vi "Slide.vi"(7 "Name (\"\" to Use UUID)":string="Event CSM") -> ()   [LabVIEW 2020]
uses:
  <userlib>/_NEVSTOP/Communicable State Machine(CSM)/AdvanceAPI/CSM - Revert Arguments-Safe String.vi
  <userlib>/_NEVSTOP/Communicable State Machine(CSM)/_Shared/Trim Single-line Text.vi
  <userlib>/_NEVSTOP/Communicable State Machine(CSM)/AdvanceAPI/CSM - Make String Arguments Safe.vi
  <userlib>/_NEVSTOP/Communicable State Machine(CSM)/AdvanceAPI/CSM - Break Down Multiple States String.vi
  <userlib>/_NEVSTOP/Communicable State Machine(CSM)/AdvanceAPI/CSM - Compact Multiple States.vi
  <userlib>/_NEVSTOP/Communicable State Machine(CSM)/AdvanceAPI/CSM - Keywords.vi
  <userlib>/_NEVSTOP/Communicable State Machine(CSM)/Communicable State Machine.lvlib
panel:
  out "Slide":u8(slide) scale=0.0..100.0
  out "State History":string
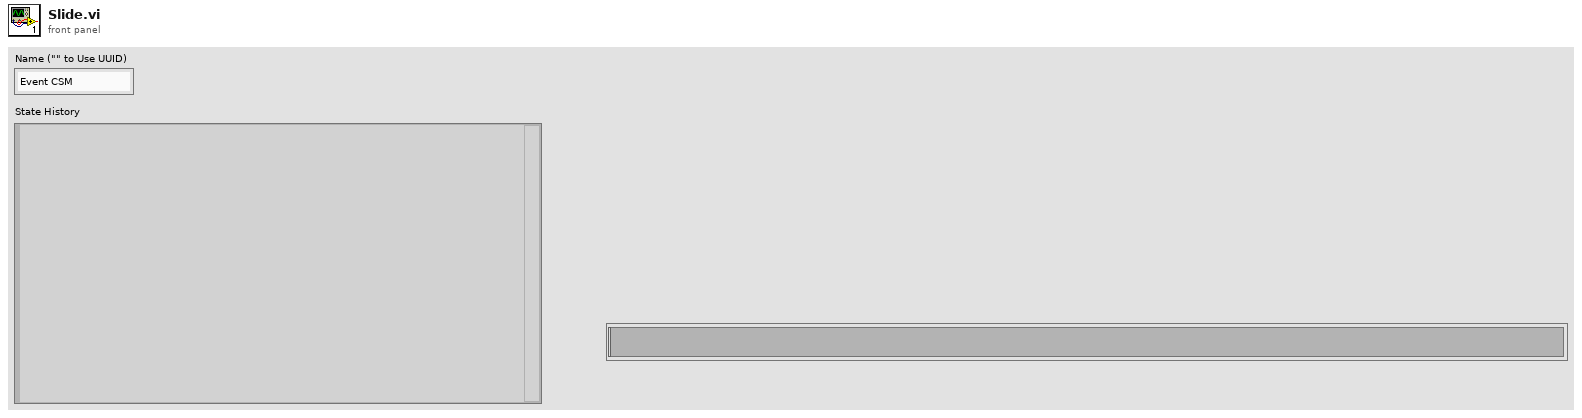
[diagram p1: front panel]
types:
  T1 = enum32{"Invalid", "Standard", "Closed", "Hidden", "Minimized", "Maximized"}
  T2 = enum32{"invalid app kind", "Development System", "Run Time System", "Student Edition", "Embedded LabVIEW", "Evaluation", "Custom"}
  T3 = typedef "Communicable State Machine.lvlib/_CSM_Response Source Message.ctl" = cluster{"‘State":string, "’Arguments":string, "’Error":errorcluster}
  T4 = cluster{"Current VI Reference":refnum<vi>, "Close Panel on Exit?":bool}
  T5 = cluster{"Core":cluster{"Current VI Reference":refnum<vi>, "Close Panel on Exit?":bool}, "Your Boolean data":bool, "Your string data":string}
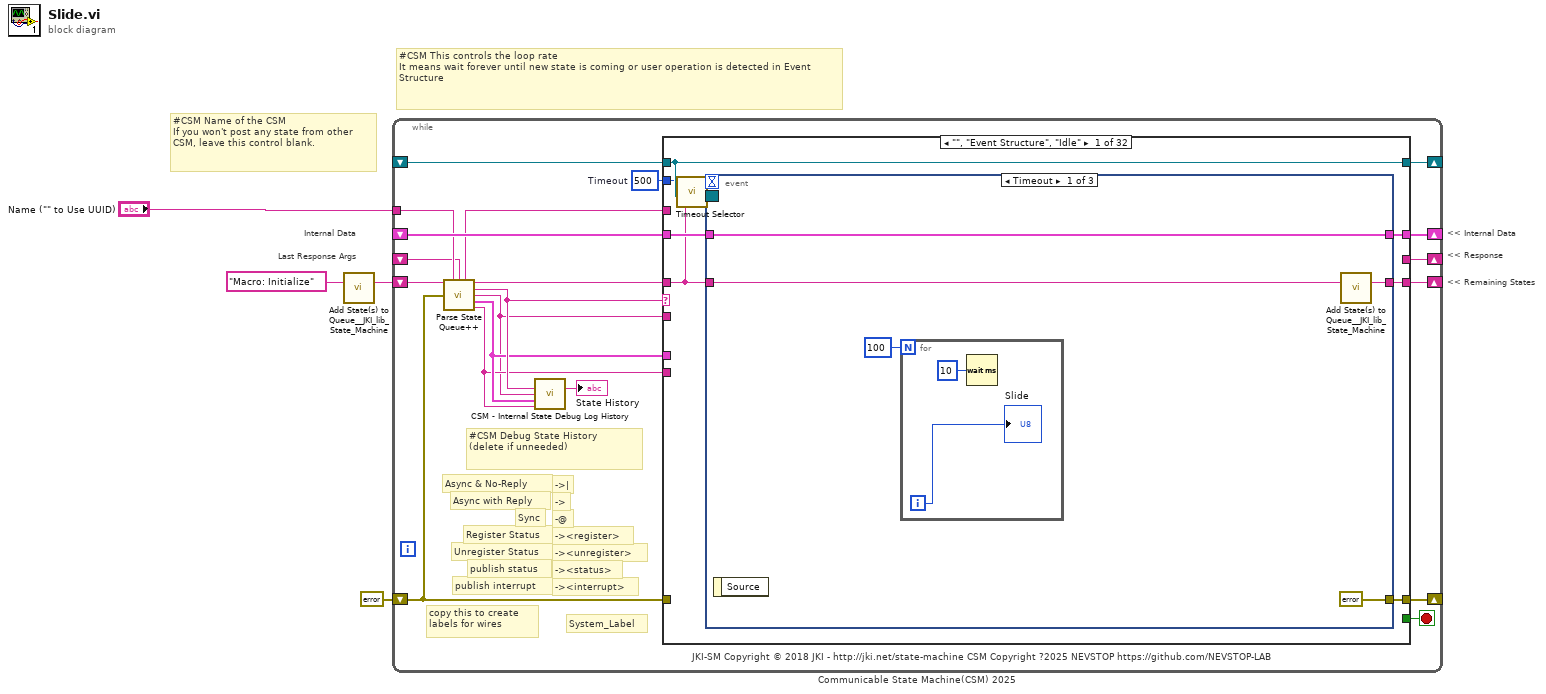
[diagram p0: block diagram]
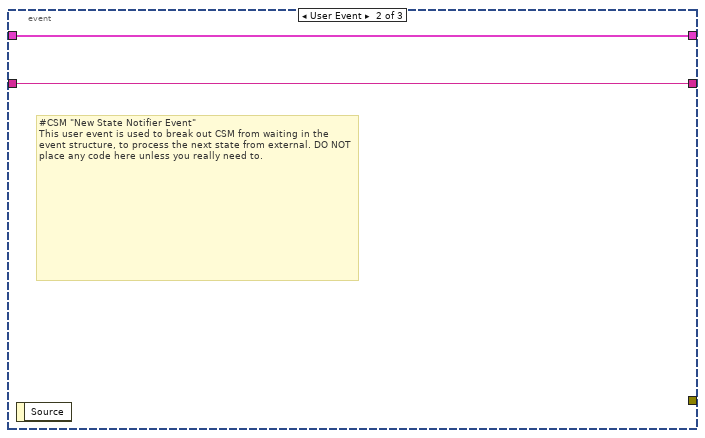
[diagram p2: hidden frame]
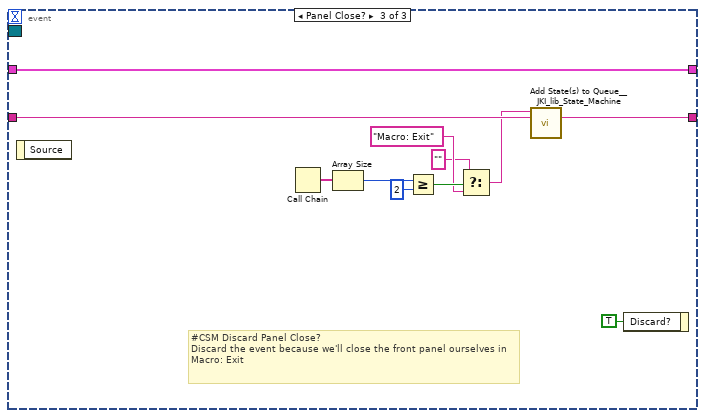
[diagram p3: hidden frame]
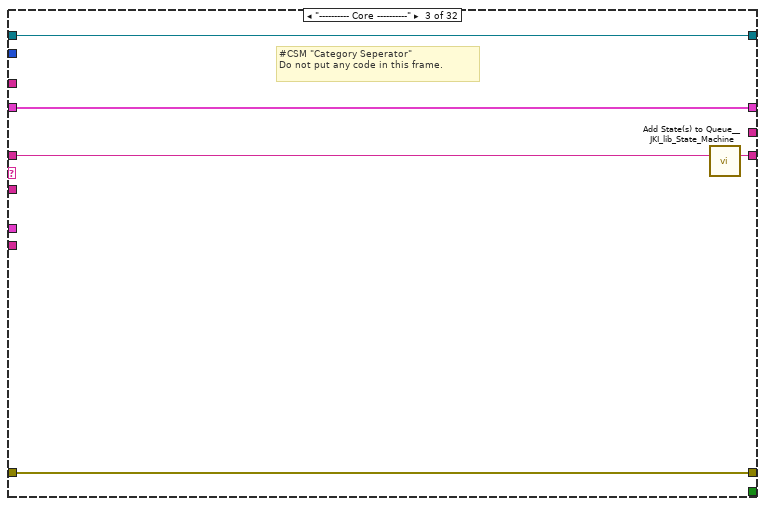
[diagram p5: hidden frame]
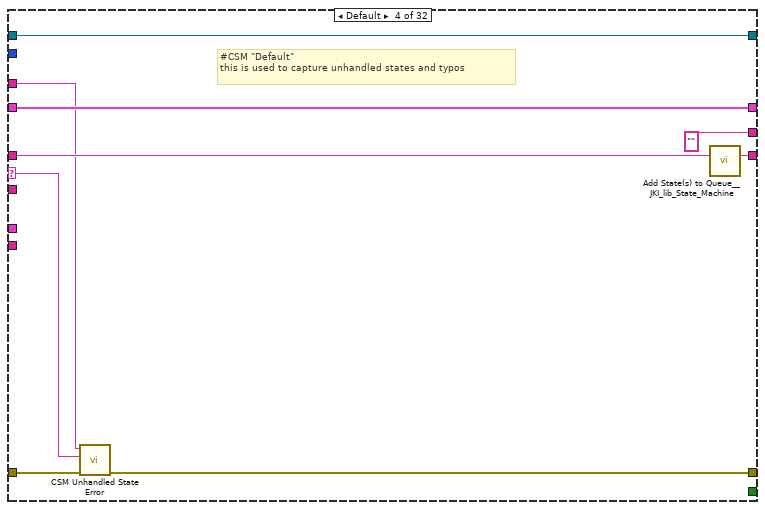
[diagram p6: hidden frame]
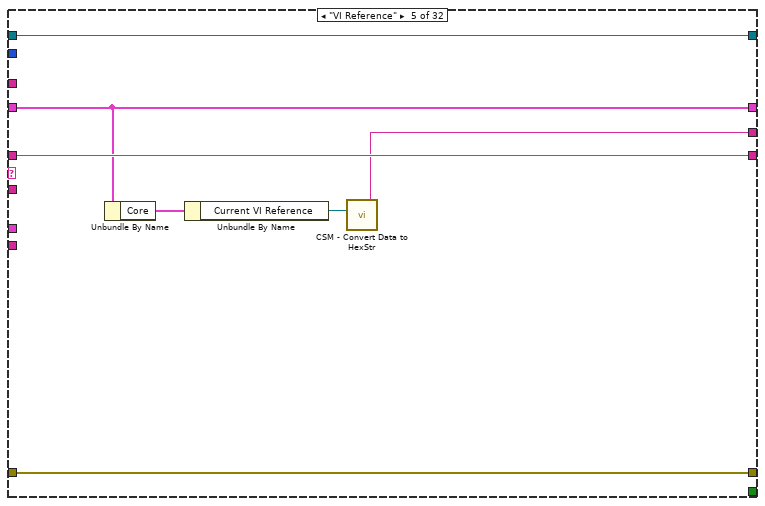
[diagram p7: hidden frame]
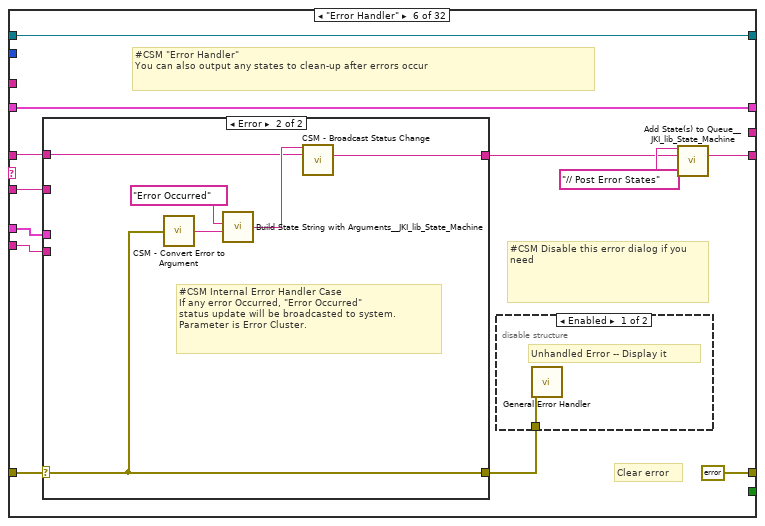
[diagram p8: hidden frame]
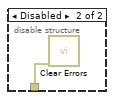
[diagram p9: hidden frame]
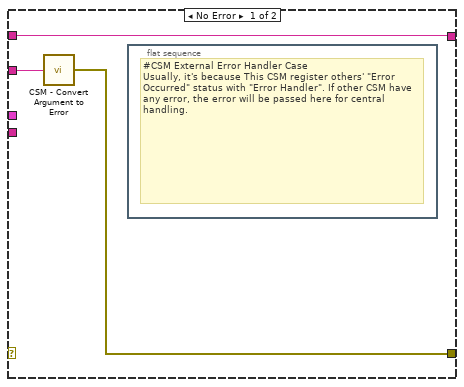
[diagram p10: hidden frame]
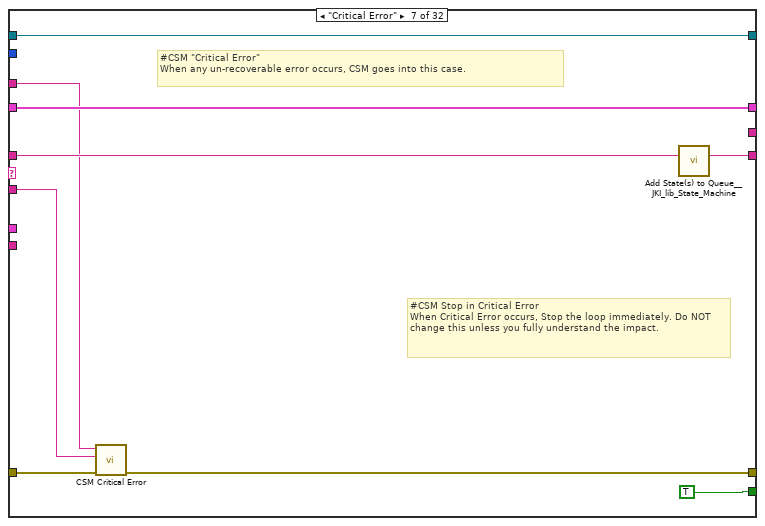
[diagram p11: hidden frame]
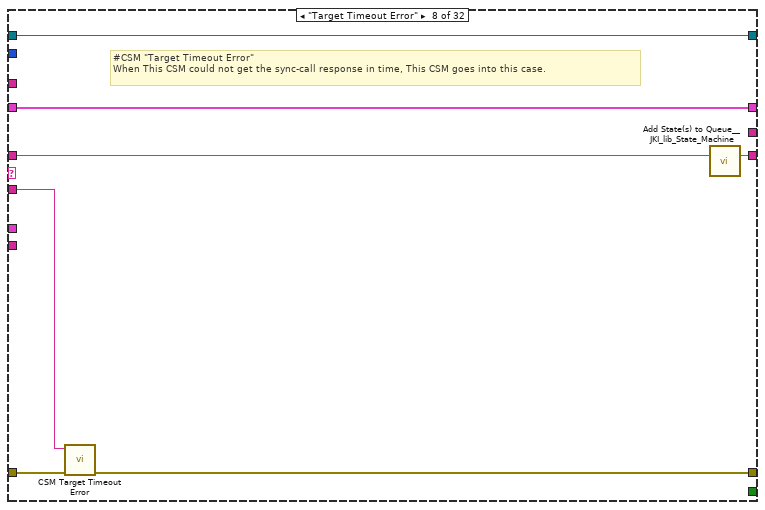
[diagram p12: hidden frame]
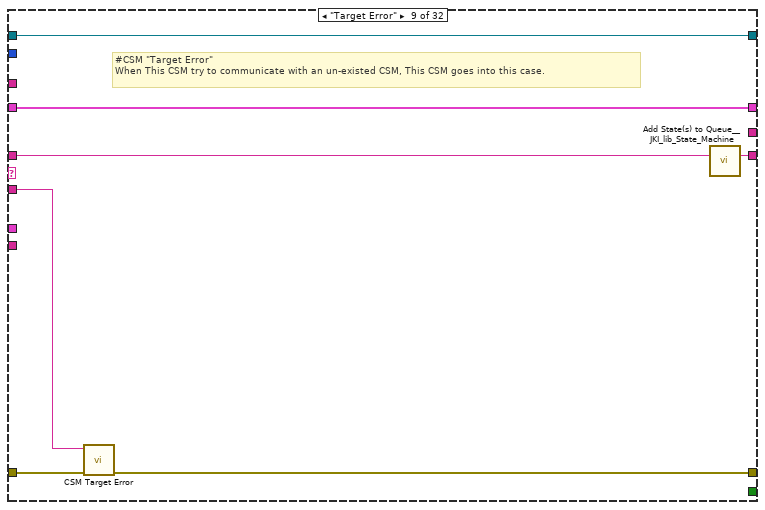
[diagram p13: hidden frame]
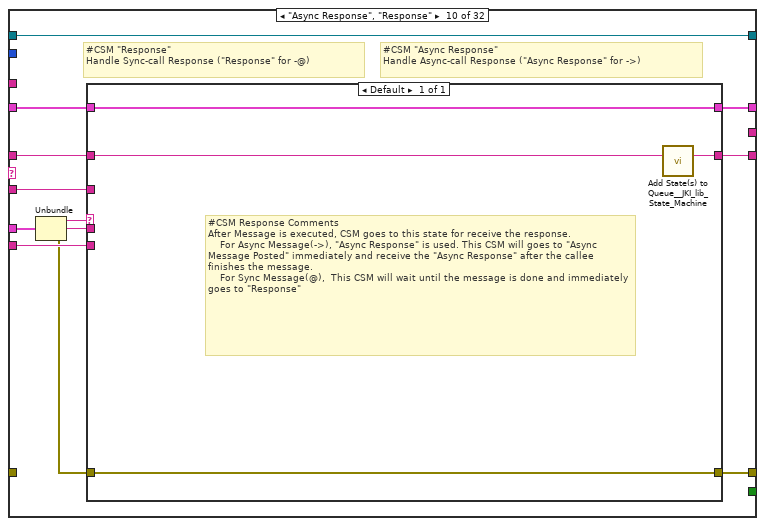
[diagram p14: hidden frame]
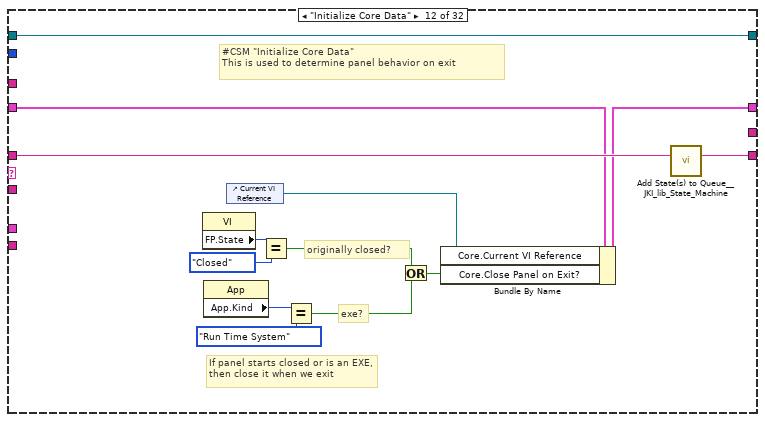
[diagram p16: hidden frame]
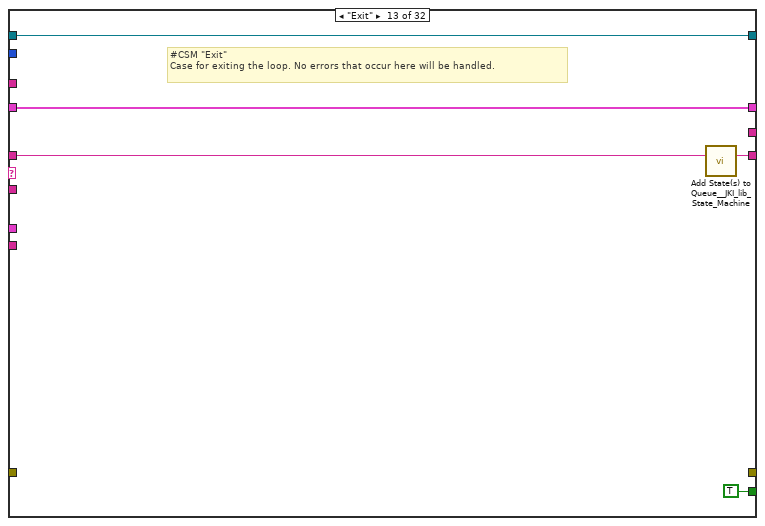
[diagram p17: hidden frame]
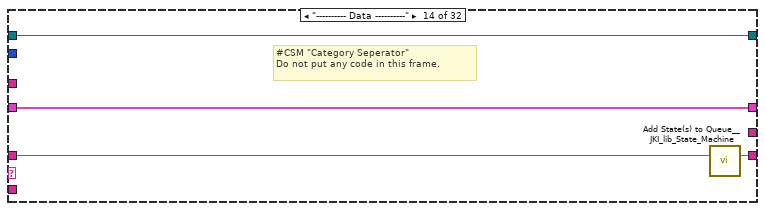
[diagram p18: hidden frame]
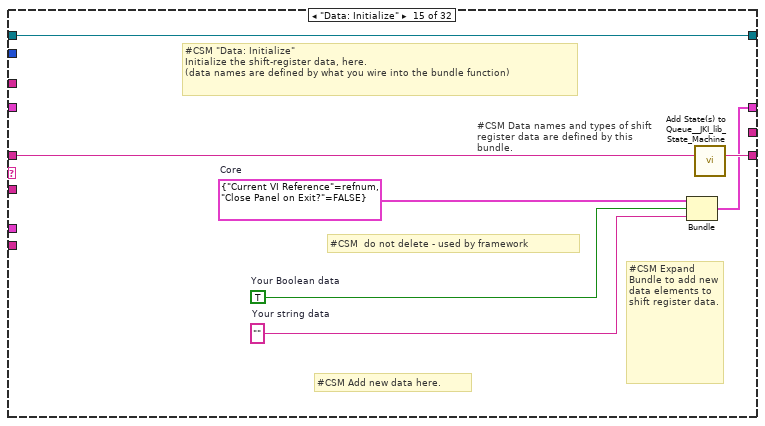
[diagram p19: hidden frame]
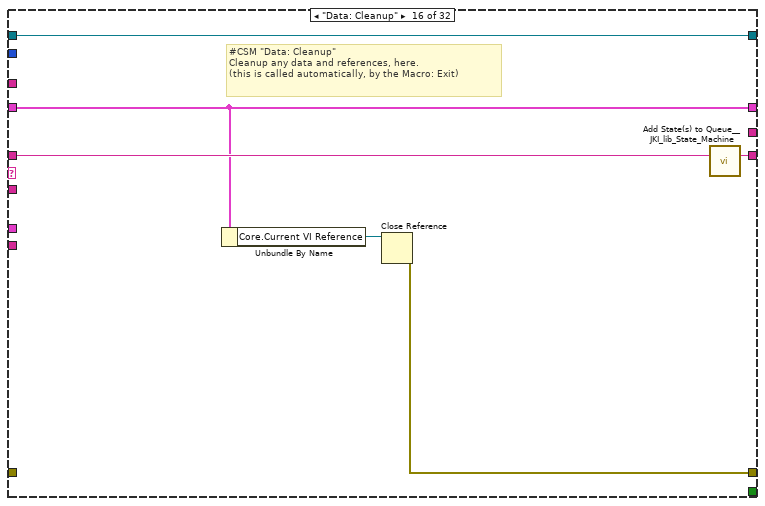
[diagram p20: hidden frame]
diagram:
  # "Last Response Args"
  # "Internal Data"
  # "<< Internal Data"
  # "<< Response"
  # "<< Remaining States"
  # "#CSM Name of the CSM\nIf you won't post any state from other CSM, leave this control blank."
  # "#CSM This controls the loop rate\nIt means wait forever until new state is coming or user operation is detected in Event Structure"
  n1 = call <vilib>:"Add State(s) to Queue__JKI_lib_State_Machine.vi"("State(s) in (\"\")"="Macro: Initialize" ("Init State(\"Macro: Initialize\")")) -> ("States Out"=w1:string)  [unwired: 14 in]
  n2 = while "Communicable State Machine(CSM) 2025" {
    shift-right: [w19] -> _
    shift-left: _ -> [w18]
    shift-right: [w22] -> _
    shift-left: errorcluster {"status"=FALSE, "code"=0, "source"=""} ("error out") -> [w16]
    shift-right: [w21] -> _
    shift-left: w1 -> [w23]
    tunnel: "Name (\"\" to Use UUID)" -> [w12]
    shift-right: [w15] -> _
    shift-left: _ -> [w7]
    shift-right: [w14] -> _
    shift-left: _ -> [w13]
    stop <- w20 stop-if-true
    w17 = 500  # Timeout
    # "#CSM Debug State History\n(delete if unneeded)"
    # "-><interrupt>"
    # "-><status>"
    # "-><unregister>"
    # "-><register>"
    # "-@"
    # "->"
    # "->|"
    # "publish interrupt"
    # "publish status"
    # "Unregister Status"
    # "Register Status"
    # "Sync"
    # "Async with Reply"
    # "Async & No-Reply"
    # "copy this to create labels for wires"
    # "System_Label"
    # "JKI-SM Copyright © 2018 JKI - http://jki.net/state-machine CSM Copyright ?2025 NEVSTOP https://github.com/NEVSTOP-LAB"
    n3 = call <userlib>:"Parse State Queue++.vi"("State Queue"=w23, "Name (\"\" to Use UUID)"=w12, "Response Arguments"=w7, "Previous Error"=w16) -> ("Name Used"=w8:string, "Remaining States"=w24:string, "Current State"=w11:string, "Arguments"=w6:string, "Additional Information"=w10:T3, "Source CSM"=w9:string)  [unwired: 6 in]
    n4 = call <userlib>:"CSM - Internal State Debug Log History.vi"("State"=w11, "Arguments (\"\")"=w6, ">> Response Source Message >>"=w10, "Source (\"\")"=w9) -> ("Debug Log"=→"State History":string)  [unwired: 11 in]
    n5 = case shown="\"\", \"Event Structure\", \"Idle\"" w11 {
      selector: w11 -> [_ _ _ w63 _ _ _ _ _ _ _ _ _ _ _ _ _ _ _ _ _ _ _ _ _ _ _ _ _ _ _ _]
      tunnel: w24 -> [w25 w55 w60 w69 w75 w81 w107 w115 w122 w132 w141 w154 w159 w163 w170 w176 w180 w187 w191 w195 w199 w205 w216 w280 w285 w296 w299 w303 w306 w310 w314 w318]
      tunnel: w6 -> [_ _ _ _ _ w79 w103 w110 w118 w126 _ _ _ _ _ _ _ _ _ _ _ w201 w211 _ _ _ _ _ _ _ _ _]
      tunnel: w18 -> [w31 w54 w57 w67 w74 w87 w108 w113 w120 w130 w140 w148 w157 w161 _ w172 w178 w186 w190 w193 w197 w203 w213 w278 w283 w294 w298 w302 w305 w308 w312 w316]
      tunnel: [w30 _ w58 w61 w76 errorcluster {"status"=FALSE, "code"=0, "source"=""} ("error out") w100 w109 w116 w129 _ _ _ _ _ w173 _ w181 w189 _ _ w202 w214 _ _ _ _ _ _ _ _ _] -> w22
      tunnel: w16 -> [_ _ w58 w62 w76 w85 w101 w111 w117 _ _ _ _ _ _ _ _ _ _ _ _ _ _ _ _ _ _ _ _ _ _ _]
      tunnel: [w32 w55 w59 w68 w75 w83 w106 w114 w121 w133 w141 w153 w158 w162 w169 w175 w179 w187 w191 w194 w198 w204 w215 w279 w284 w295 w299 w303 w306 w309 w313 w317] -> w21
      tunnel: [_ _ _ _ _ _ TRUE _ _ _ _ _ TRUE _ _ _ _ _ _ _ _ _ _ _ _ _ _ _ _ _ _ _] -> w20
      tunnel: [w29 w54 w57 w67 w74 w87 w108 w113 w120 w131 w140 w152 w157 w161 w168 w172 w178 w186 w190 w193 w197 w203 w213 w278 w283 w294 w298 w302 w305 w308 w312 w316] -> w19
      tunnel: w17 -> [w27 _ _ _ _ _ _ _ _ _ _ _ _ _ _ _ _ _ _ _ _ _ _ _ _ _ _ _ _ _ _ _]
      tunnel: w9 -> [_ _ _ _ _ w78 _ _ _ w127 _ _ _ _ _ _ _ _ _ _ _ _ _ _ _ _ _ _ _ _ _ _]
      tunnel: w10 -> [_ _ _ _ _ w77 _ _ _ w128 _ _ _ _ _ _ _ _ _ _ _ _ _ _ _ _ _ _ _ _ _ _]
      tunnel: [_ _ _ "" w70 _ _ _ _ _ _ _ _ _ _ _ _ _ _ _ _ _ _ _ _ _ _ "API1 Response" _ _ _ _] -> w15
      tunnel: [w28 w53 w56 w65 w73 w86 w104 w112 w119 w134 w139 w142 w155 w160 w164 w171 w177 w185 w188 w192 w196 w200 w210 w277 w281 w287 w297 w301 w304 w307 w311 w315] -> w14
      tunnel: w13 -> [w28 w53 w56 w65 w73 w86 w104 w112 w119 w134 w139 w142 w155 w160 w164 w171 w177 _ w188 w192 w196 w200 w210 w277 w281 w287 w297 w301 w304 w307 w311 w315]
      tunnel: w8 -> [_ _ _ w64 _ _ w102 _ _ _ _ _ _ _ _ _ _ w184 _ _ _ _ _ _ _ _ _ _ _ _ _ _]
      frame "", "Event Structure", "Idle" {
        n6 = call <userlib>:"Timeout Selector.vi"("Remaining States"=w25, "Timeout Expected"=w27) -> ("Timeout"=w26:i32)  [unwired: 5 in]
        n7 = event shown="[0] Timeout" {
          selector: w28 -> [_ _ _]
          dyn-events: _ -> [_ _ _]
          timeout: w26 -> [_ _ _]
          tunnel: w25 -> [w37 w40 w52]
          tunnel: [w36 w40 w51] -> w32
          tunnel: w31 -> [w35 w41 w50]
          tunnel: [errorcluster {"status"=FALSE, "code"=0, "source"=""} ("error out") _ _] -> w30
          tunnel: [w35 w41 w50] -> w29
          event Timeout {
            n8 = event-data() -> ()  [unwired: 1 in, 1 out]
            n9 = for {
              N: 100 -> [_]
              i -> [w39]
              n10 = Wait (ms)(milliseconds to wait=u32 10) -> ()  [unwired: 1 out]
              "Slide" <- w39
            }
            n11 = call <vilib>:"Add State(s) to Queue__JKI_lib_State_Machine.vi"("State(s) in (\"\")"=w37) -> ("States Out"=w36:string)  [unwired: 14 in]
          }
          event User Event {
            # "#CSM \"New State Notifier Event\"\nThis user event is used to break out CSM from waiting in the event structure, to process the next state from external. DO NOT place any code here unless you really need to."
            n12 = event-data() -> ()  [unwired: 1 in, 1 out]
          }
          event Panel Close? {
            # "#CSM Discard Panel Close?\nDiscard the event because we'll close the front panel ourselves in Macro: Exit"
            n13 = event-data() -> ()  [unwired: 1 in, 1 out]
            n14 = Call Chain() -> (call chain=w42:string[])
            n15 = Array Size(array=w42) -> (size(s)=w48:i32)
            n16 = Greater Or Equal?(x=w48, y=2) -> (x >= y?=w46:bool)
            n17 = Select(t="", s=w46, f="Macro: Exit") -> (s? t:f=w43:string)
            n18 = call <vilib>:"Add State(s) to Queue__JKI_lib_State_Machine.vi"("State(s) in Front (\"\")"=w43, "State(s) in (\"\")"=w52) -> ("States Out"=w51:string)  [unwired: 13 in]
            n19 = event-data("Discard?"=TRUE) -> ()  [unwired: 1 in, 1 out]
          }
        }
      }
      frame "CSM Documentation" {
        # "#CSM State Syntax\n\n// Comment line, all text to the right of “//” will be ignored\n// Local Message Example\nDoSth: DoA >> Arguments\n\n// Sync Call Example\nAPI: xxxx >> Arguments -@ TargetModule\n\n// Async Call Example\nAPI: xxxx >> Arguments -> TargetModule\n\n// Async Call without Reply Example\nAPI: xxxx >> Arguments ->| TargetModule\n\n// Broadcast normal status:\nStatus >> StatusArguments  -><status>\n\n// Broadcast Interrupt status:\nInterrupt >> StatusArguments  -><interrupt>\n\n// Register Source Module's status to Handler Module\nStatus@Source Module >> Handler Module@Handler Module -><register>\n\n// Unegister Source Module's status\nStatus@Source Module >> Handler Module -><unregister>"
        # "#CSM README FIRST\n\nCommunicable State Machine(CSM) is a LabVIEW application framework that builds upon JKI State Machine(JKISM). It follows the pattern of JKISM and extends the keywords to describe message communication between modules, including concepts such as Sync-Message, Async-Message, Subscription/Unsubscription of status - essential elements for creating reusable code modules. For more information, please visit the CSM wiki: https://nevstop-lab.github.io/CSM-Wiki/\n\nFor instructions on JKI State Machine, visit: \n    http://jki.net/state-machine/\nFor information about CSM, visit: \n    https://github.com/NEVSTOP-LAB"
        # "#CSM \"Documentation\"\nCase for holding CSM Documenation"
      }
      frame "---------- Core ----------" {
        # "#CSM \"Category Seperator\"\nDo not put any code in this frame."
        n20 = call <vilib>:"Add State(s) to Queue__JKI_lib_State_Machine.vi"("State(s) in (\"\")"=w60) -> ("States Out"=w59:string)  [unwired: 14 in]
      }
      frame Default {
        # "#CSM \"Default\"\nthis is used to capture unhandled states and typos"
        n21 = call <userlib>:"CSM Unhandled State Error.vi"("error in (no error)"=w62, "Undefined State"=w63, "CSM Name"=w64) -> ("error out"=w61:errorcluster)  [unwired: 8 in]
        n22 = call <vilib>:"Add State(s) to Queue__JKI_lib_State_Machine.vi"("State(s) in (\"\")"=w69) -> ("States Out"=w68:string)  [unwired: 14 in]
      }
      frame "VI Reference" {
        n23 = Unbundle By Name(w74) -> ("Core"=w72:T4)
        n24 = Unbundle By Name(w72) -> ("Current VI Reference"=w71:refnum<vi>)
        n25 = call <userlib>:"CSM - Convert Data to HexStr.vi"("Variant"=w71) -> ("HEX String (0-9,A-F)"=w70:string)  [unwired: 8 in]
      }
      frame "Error Handler" {
        # "#CSM Disable this error dialog if you need"
        # "#CSM \"Error Handler\"\nYou can also output any states to clean-up after errors occur"
        # "Clear error"
        n26 = case shown="Error" w85 {
          selector: w85 -> [_ w94]
          tunnel: [w92 w96] -> w82
          tunnel: w81 -> [w92 w95]
          tunnel: [w91 w94] -> w80
          tunnel: w79 -> [w93 _]
          tunnel: w78 -> [_ _]
          tunnel: w77 -> [_ _]
          frame No Error {
            n27 = call <userlib>:"CSM - Convert Argument to Error.vi"("Argument"=w93) -> ("Error"=w91:errorcluster)  [unwired: 4 in]
            n28 = flat-sequence {
              frame #0 {
                # "#CSM External Error Handler Case\nUsually, it's because This CSM register others' \"Error Occurred\" status with \"Error Handler\". If other CSM have any error, the error will be passed here for central handling."
              }
            }
          }
          frame Error {
            # "#CSM Internal Error Handler Case \nIf any error Occurred, \"Error Occurred\" \nstatus update will be broadcasted to system.\nParameter is Error Cluster."
            n29 = call <userlib>:"CSM - Convert Error to Argument.vi"("Error"=w94) -> ("Argument"=w98:string)  [unwired: 4 in]
            n30 = call <vilib>:"Build State String with Arguments__JKI_lib_State_Machine.vi"("Arguments (\"\")"=w98, "State"="Error Occurred" ("Status with Arguments")) -> ("State with Arguments"=w97:string)  [unwired: 4 in]
            n31 = call <userlib>:"CSM - Broadcast Status Change.vi"("Status With Arguments"=w97, "State Queue"=w95) -> ("Remaining States"=w96:string)  [unwired: 13 in]
          }
        }
        n32 = disable-structure shown="Enabled" {
          disable-tunnel: w80 -> [w89 w90]
          frame Enabled {
            # "Unhandled Error -- Display it"
            n33 = call <vilib>:"General Error Handler.vi"("error in (no error)"=w89) -> ()  [unwired: 10 in, 5 out]
          }
          frame Disabled {
            n34 = call <vilib>:"Clear Errors.vi"("error in (no error)"=w90) -> ()  [unwired: 5 in, 2 out]
          }
        }
        n35 = call <vilib>:"Add State(s) to Queue__JKI_lib_State_Machine.vi"("State(s) in Front (\"\")"="// Post Error States", "State(s) in (\"\")"=w82) -> ("States Out"=w83:string)  [unwired: 13 in]
      }
      frame "Critical Error" {
        # "#CSM \"Critical Error\"\nWhen any un-recoverable error occurs, CSM goes into this case."
        # "#CSM Stop in Critical Error\nWhen Critical Error occurs, Stop the loop immediately. Do NOT change this unless you fully understand the impact."
        n36 = call <userlib>:"CSM Critical Error.vi"("error in (no error)"=w101, "Arugments (As Reason)"=w103, "CSM Name"=w102) -> ("error out"=w100:errorcluster)  [unwired: 8 in]
        n37 = call <vilib>:"Add State(s) to Queue__JKI_lib_State_Machine.vi"("State(s) in (\"\")"=w107) -> ("States Out"=w106:string)  [unwired: 14 in]
      }
      frame "Target Timeout Error" {
        # "#CSM \"Target Timeout Error\"\nWhen This CSM could not get the sync-call response in time, This CSM goes into this case."
        n38 = call <userlib>:"CSM Target Timeout Error.vi"("error in (no error)"=w111, "Arguments (As CSM Name)"=w110) -> ("error out"=w109:errorcluster)  [unwired: 9 in]
        n39 = call <vilib>:"Add State(s) to Queue__JKI_lib_State_Machine.vi"("State(s) in (\"\")"=w115) -> ("States Out"=w114:string)  [unwired: 14 in]
      }
      frame "Target Error" {
        # "#CSM \"Target Error\"\nWhen This CSM try to communicate with an un-existed CSM, This CSM goes into this case."
        n40 = call <userlib>:"CSM Target Error.vi"("error in (no error)"=w117, "Arguments (As CSM Name)"=w118) -> ("error out"=w116:errorcluster)  [unwired: 9 in]
        n41 = call <vilib>:"Add State(s) to Queue__JKI_lib_State_Machine.vi"("State(s) in (\"\")"=w122) -> ("States Out"=w121:string)  [unwired: 14 in]
      }
      frame "Async Response", "Response" {
        # "#CSM \"Async Response\"\nHandle Async-call Response (\"Async Response\" for ->)"
        # "#CSM \"Response\"\nHandle Sync-call Response (\"Response\" for -@)"
        n42 = Unbundle(w128) -> ("‘State"=w125:string, "’Arguments"=w124:string, "’Error"=w123:errorcluster)
        n43 = case shown="Default" w125 {
          tunnel: [w135] -> w133
          tunnel: w132 -> [w136]
          tunnel: [w138] -> w131
          tunnel: w130 -> [w138]
          tunnel: [w137] -> w129
          tunnel: w123 -> [w137]
          tunnel: w127 -> [_]
          tunnel: w126 -> [_]
          tunnel: w124 -> [_]
          frame Default {
            # "#CSM Response Comments\nAfter Message is executed, CSM goes to this state for receive the response.\n    For Async Message(->), \"Async Response\" is used. This CSM will goes to \"Async Message Posted\" immediately and receive the \"Async Response\" after the callee finishes the message.\n    For Sync Message(@),  This CSM will wait until the message is done and immediately goes to \"Response\""
            n44 = call <vilib>:"Add State(s) to Queue__JKI_lib_State_Machine.vi"("State(s) in (\"\")"=w136) -> ("States Out"=w135:string)  [unwired: 14 in]
          }
        }
      }
      frame "Async Message Posted" {
        # "#CSM \"Async Message Posted\"\nAfter Async Message is posted (-> or ->| ), CSM goes to this state for post-action.\nYou can use Argument - State to tell which Async Message is called."
      }
      frame "Initialize Core Data" {
        # "#CSM \"Initialize Core Data\"\nThis is used to determine panel behavior on exit"
        # "originally closed?"
        # "exe?"
        # "If panel starts closed or is an EXE, then close it when we exit"
        n45 = property class="VI"() -> ("FP.State"=w145:T1)  [unwired: 2 in, 2 out]
        n46 = property class="App"() -> ("App.Kind"=w151:T2)  [unwired: 2 in, 2 out]
        n47 = control-ref of="Current VI Reference"() -> (w146:refnum<vi>)
        n48 = Equal?(x=w145, y=T1."Closed" ("Front Panel Window:State")) -> (x = y?=w143:bool)
        n49 = Equal?(x=w151, y=T2."Run Time System" ("Application:Kind")) -> (x = y?=w149:bool)
        n50 = Or(x=w143, y=w149) -> (x .or. y?=w147:bool)
        n51 = Bundle By Name(cluster=w148, "Core.Current VI Reference"=w146, "Core.Close Panel on Exit?"=w147) -> (w152:T5)
        n52 = call <vilib>:"Add State(s) to Queue__JKI_lib_State_Machine.vi"("State(s) in (\"\")"=w154) -> ("States Out"=w153:string)  [unwired: 14 in]
      }
      frame "Exit" {
        # "#CSM \"Exit\"\nCase for exiting the loop. No errors that occur here will be handled."
        n53 = call <vilib>:"Add State(s) to Queue__JKI_lib_State_Machine.vi"("State(s) in (\"\")"=w159) -> ("States Out"=w158:string)  [unwired: 14 in]
      }
      frame "---------- Data ----------" {
        # "#CSM \"Category Seperator\"\nDo not put any code in this frame."
        n54 = call <vilib>:"Add State(s) to Queue__JKI_lib_State_Machine.vi"("State(s) in (\"\")"=w163) -> ("States Out"=w162:string)  [unwired: 14 in]
      }
      frame "Data: Initialize" {
        w165 = T4 {"Current VI Reference"=refnum, "Close Panel on Exit?"=FALSE}  # Core
        w167 = TRUE  # Your Boolean data
        w166 = ""  # Your string data
        # "#CSM  do not delete - used by framework"
        # "#CSM Expand Bundle to add new data elements to shift register data."
        # "#CSM Add new data here."
        # "#CSM Data names and types of shift register data are defined by this bundle."
        # "#CSM \"Data: Initialize\"\nInitialize the shift-register data, here.\n(data names are defined by what you wire into the bundle function)"
        n55 = Bundle("Core"=w165, "Your Boolean data"=w167, "Your string data"=w166) -> (w168:T5)  [unwired: 1 in]
        n56 = call <vilib>:"Add State(s) to Queue__JKI_lib_State_Machine.vi"("State(s) in (\"\")"=w170) -> ("States Out"=w169:string)  [unwired: 14 in]
      }
      frame "Data: Cleanup" {
        # "#CSM \"Data: Cleanup\"\nCleanup any data and references, here.\n(this is called automatically, by the Macro: Exit)"
        n57 = Unbundle By Name(w172) -> ("Core.Current VI Reference"=w174:refnum<vi>)
        n58 = Close Reference(reference=w174) -> (error out=w173:errorcluster)  [unwired: 1 in]
        n59 = call <vilib>:"Add State(s) to Queue__JKI_lib_State_Machine.vi"("State(s) in (\"\")"=w176) -> ("States Out"=w175:string)  [unwired: 14 in]
      }
      frame "---------- Events ----------" {
        # "#CSM \"Category Seperator\"\nDo not put any code in this frame."
        n60 = call <vilib>:"Add State(s) to Queue__JKI_lib_State_Machine.vi"("State(s) in (\"\")"=w180) -> ("States Out"=w179:string)  [unwired: 14 in]
      }
      frame "Events: Register" {
        # "#CSM \"Events: Register\"\nRegister user event. New Message Event is registered to break CSM waiting in event structure by default."
        # "#CSM Register New Message Event\nRegister message event to break Waiting in Event structure."
        n61 = call <userlib>:"CSM - Get New State Notifier Event.vi"("Name (\"\" to Use UUID)"=w184) -> ("error out"=w182:errorcluster, "New State Notifier Event"=w183:refnum<user-event>)  [unwired: 9 in]
        n62 = register-events(error in=w182, w183) -> (reference out=w185:refnum<event-registration>, error out=w181:errorcluster)  [unwired: 1 in]
      }
      frame "Events: Unregister" {
        # "#CSM \"Events: Unregister\"\nUnregister user event."
        n63 = Unregister For Events(event registration refnum=w188) -> (error out=w189:errorcluster)  [unwired: 1 in]
      }
      frame "---------- UI ----------" {
        # "#CSM \"Category Seperator\"\nDo not put any code in this frame."
        n64 = call <vilib>:"Add State(s) to Queue__JKI_lib_State_Machine.vi"("State(s) in (\"\")"=w195) -> ("States Out"=w194:string)  [unwired: 14 in]
      }
      frame "UI: Initialize" {
        # "#CSM \"UI: Initialize\"\nInitialize the User Interface, here.\n(this is called automatically, by the Macro: Init)"
        n65 = call <vilib>:"Add State(s) to Queue__JKI_lib_State_Machine.vi"("State(s) in (\"\")"=w199) -> ("States Out"=w198:string)  [unwired: 14 in]
      }
      frame "UI: Cursor Set" {
        # "Argument"
        # "#CSM \"UI: Cursor Set\"\nSet and Unset Cursor Busy.\n(Usage: \"UI: Cursor Set >> Busy|Idle\")"
        n66 = disable-structure shown="TARGET_TYPE!=Windows" {
          disable-tunnel: [w207 _] -> w202
          disable-tunnel: w201 -> [w206 _]
          frame condition #0 (active) {
            n67 = case shown="\"Idle\", Default" w206 {
              tunnel: [w208 w209] -> w207
              frame "Idle", Default {
                n68 = call <vilib>:"Unset Busy.vi"() -> ("error out"=w208:errorcluster)  [unwired: 11 in]
              }
              frame "Busy" {
                n69 = call <vilib>:"Set Busy.vi"() -> ("error out"=w209:errorcluster)  [unwired: 10 in, 1 out]
              }
            }
          }
          frame condition #1 {
          }
        }
        n70 = call <vilib>:"Add State(s) to Queue__JKI_lib_State_Machine.vi"("State(s) in (\"\")"=w205) -> ("States Out"=w204:string)  [unwired: 14 in]
      }
      frame "UI: Front Panel State" {
        # "Argument"
        # "#CSM \"UI: Front Panel State\"\nSet Front Panel Open or Closed\n(Usage: \"UI: Front Panel State >> Open|Close\")"
        n71 = Unbundle By Name(w213) -> ("Core.Current VI Reference"=w212:refnum<vi>)
        n72 = case shown="\"Open\", \"Standard\", Default" w211 {
          tunnel: [w223 w236 w247 w259 w271] -> w214
          tunnel: w212 -> [w222 w234 w246 w258 w270]
          frame "Open", "Standard", Default {
            w217 = T1."Standard" ("State")
            n73 = property class="VI"(reference=w222) -> (reference out=w220:refnum<vi>, error out=w221:errorcluster, "FP.State"=w219:T1)  [unwired: 1 in]
            n74 = Not Equal?(x=w219, y=w217) -> (x != y?=w218:bool)
            n75 = case shown="True" w218 {
              tunnel: [w227 w229] -> w223
              tunnel: w221 -> [w226 w229]
              tunnel: w220 -> [w225 _]
              tunnel: w217 -> [w224 _]
              frame True {
                n76 = invoke class="VI" method="FP.Open"(reference=w225, error in=w226, "Activate"=TRUE, "State"=w224) -> (error out=w227:errorcluster)  [unwired: 1 in, 4 out]
              }
              frame False {
              }
            }
          }
          frame "Close", "Closed" {
            n77 = property class="VI"(reference=w234) -> (reference out=w233:refnum<vi>, error out=w235:errorcluster, "FP.State"=w231:T1)  [unwired: 1 in]
            n78 = Not Equal?(x=w231, y=T1."Closed" ("Front Panel Window:State")) -> (x != y?=w230:bool)
            n79 = case shown="True" w230 {
              tunnel: [w237 w240] -> w236
              tunnel: w235 -> [w237 w239]
              tunnel: w233 -> [_ w238]
              frame False {
              }
              frame True {
                n80 = invoke class="VI" method="FP.Close"(reference=w238, error in=w239) -> (error out=w240:errorcluster)  [unwired: 1 in, 2 out]
              }
            }
          }
          frame "Hidden", "Hide" {
            w241 = T1."Hidden" ("State")
            n81 = property class="VI"(reference=w246) -> (reference out=w244:refnum<vi>, error out=w245:errorcluster, "FP.State"=w243:T1)  [unwired: 1 in]
            n82 = Not Equal?(x=w243, y=w241) -> (x != y?=w242:bool)
            n83 = case shown="True" w242 {
              tunnel: [w251 w252] -> w247
              tunnel: w245 -> [w250 w252]
              tunnel: w244 -> [w249 _]
              tunnel: w241 -> [w248 _]
              frame True {
                n84 = invoke class="VI" method="FP.Open"(reference=w249, error in=w250, "State"=w248) -> (error out=w251:errorcluster)  [unwired: 2 in, 4 out]
              }
              frame False {
              }
            }
          }
          frame "Minimize", "Minimized" {
            w253 = T1."Minimized" ("State")
            n85 = property class="VI"(reference=w258) -> (reference out=w256:refnum<vi>, error out=w257:errorcluster, "FP.State"=w255:T1)  [unwired: 1 in]
            n86 = Not Equal?(x=w255, y=w253) -> (x != y?=w254:bool)
            n87 = case shown="False" w254 {
              tunnel: [w263 w264] -> w259
              tunnel: w257 -> [w262 w264]
              tunnel: w256 -> [w261 _]
              tunnel: w253 -> [w260 _]
              frame True {
                n88 = invoke class="VI" method="FP.Open"(reference=w261, error in=w262, "State"=w260) -> (error out=w263:errorcluster)  [unwired: 2 in, 4 out]
              }
              frame False {
              }
            }
          }
          frame "Maximize", "Maximized" {
            w265 = T1."Maximized" ("State")
            n89 = property class="VI"(reference=w270) -> (reference out=w268:refnum<vi>, error out=w269:errorcluster, "FP.State"=w267:T1)  [unwired: 1 in]
            n90 = Not Equal?(x=w267, y=w265) -> (x != y?=w266:bool)
            n91 = case shown="True" w266 {
              tunnel: [w275 w276] -> w271
              tunnel: w269 -> [w274 w276]
              tunnel: w268 -> [w273 _]
              tunnel: w265 -> [w272 _]
              frame True {
                n92 = invoke class="VI" method="FP.Open"(reference=w273, error in=w274, "State"=w272) -> (error out=w275:errorcluster)  [unwired: 2 in, 4 out]
              }
              frame False {
              }
            }
          }
        }
        n93 = call <vilib>:"Add State(s) to Queue__JKI_lib_State_Machine.vi"("State(s) in (\"\")"=w216) -> ("States Out"=w215:string)  [unwired: 14 in]
      }
      frame "---------- Macro ----------" {
        # "#CSM \"Category Seperator\"\nDo not put any code in this frame."
        n94 = call <vilib>:"Add State(s) to Queue__JKI_lib_State_Machine.vi"("State(s) in (\"\")"=w280) -> ("States Out"=w279:string)  [unwired: 14 in]
      }
      frame "Macro: Initialize" {
        w282 = "Data: Initialize\nInitialize Core Data\nEvents: Register\nUI: Initialize\n//UI: Front Panel State >> Open"  # Data: Initialize Initialize Core Data Events: Register UI: Initialize //UI: Front Panel State >> Open
        # "#CSM \"Macro: Initialize\"\nInitialization Macro (This is called once, when the VI starts)"
        n95 = call <vilib>:"Add State(s) to Queue__JKI_lib_State_Machine.vi"("State(s) in Front (\"\")"=w282, "State(s) in (\"\")"=w285) -> ("States Out"=w284:string)  [unwired: 13 in]
      }
      frame "Macro: Exit" {
        # "#CSM \"Macro: Exit\"\nExit Macro (This is called once, when the VI exits)"
        n96 = Unbundle By Name(w294) -> ("Core.Close Panel on Exit?"=w293:bool)
        n97 = Select(t="UI: Front Panel State >> Close", s=w293, f="") -> (s? t:f=w290:string)
        n98 = call <vilib>:"Add State(s) to Queue__JKI_lib_State_Machine.vi"("State(s) in Front (\"\")"="//Exit Sub-Modules ", "State(s) in (\"\")"=w290, "State(s) at Back (\"\")"="Data: Cleanup\nEvents: Unregister\nExit") -> ("States Out"=w288:string)  [unwired: 12 in]
        n99 = call <vilib>:"Add State(s) to Queue__JKI_lib_State_Machine.vi"("State(s) in Front (\"\")"=w288, "State(s) in (\"\")"=w296) -> ("States Out"=w295:string)  [unwired: 13 in]
      }
      frame "---------- API ----------" {
        # "#CSM \"Category Seperator\"\nDo not put any code in this frame."
      }
      frame "API: API1" {
        # "#CSM >> Source CSM >>\nIf you need to tell who triggered this state , use this string. If it's this case itself, this string is \"\"."
        # "#CSM >> Arguments >>\nDeal with the parameter if any"
        # "#CSM Response\nConnect this to return the response of your API"
        # "#CSM API Example\nCopy/Rename this case for your own API"
      }
      frame "API: API2" {
        # "#CSM API Example\nCopy/Rename this case for your own API"
      }
      frame "---------- Action ----------" {
        # "#CSM \"Category Seperator\"\nDo not put any code in this frame."
        n100 = call <vilib>:"Add State(s) to Queue__JKI_lib_State_Machine.vi"("State(s) in (\"\")"=w310) -> ("States Out"=w309:string)  [unwired: 14 in]
      }
      frame "Action: action1" {
        # "#CSM \"Internal State\"\nThis category is used for holding internal states"
        n101 = call <vilib>:"Add State(s) to Queue__JKI_lib_State_Machine.vi"("State(s) in (\"\")"=w314) -> ("States Out"=w313:string)  [unwired: 14 in]
      }
      frame "Action: action2" {
        # "#CSM \"Internal State\"\nThis category is used for holding internal states"
        n102 = call <vilib>:"Add State(s) to Queue__JKI_lib_State_Machine.vi"("State(s) in (\"\")"=w318) -> ("States Out"=w317:string)  [unwired: 14 in]
      }
    }
  }
